vi "Entanglement Table - Read.vi"(7 "QuWire in":refnum<class "QuWire.lvclass">) -> (8 "Mutal Information Table":dbl[][](array[numeric]))   [LabVIEW 2020]
uses:
  QuSim/QuWire/QuWire.lvclass
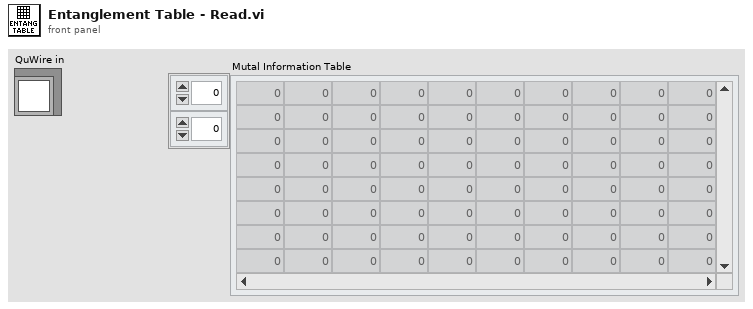
[diagram p1: front panel]
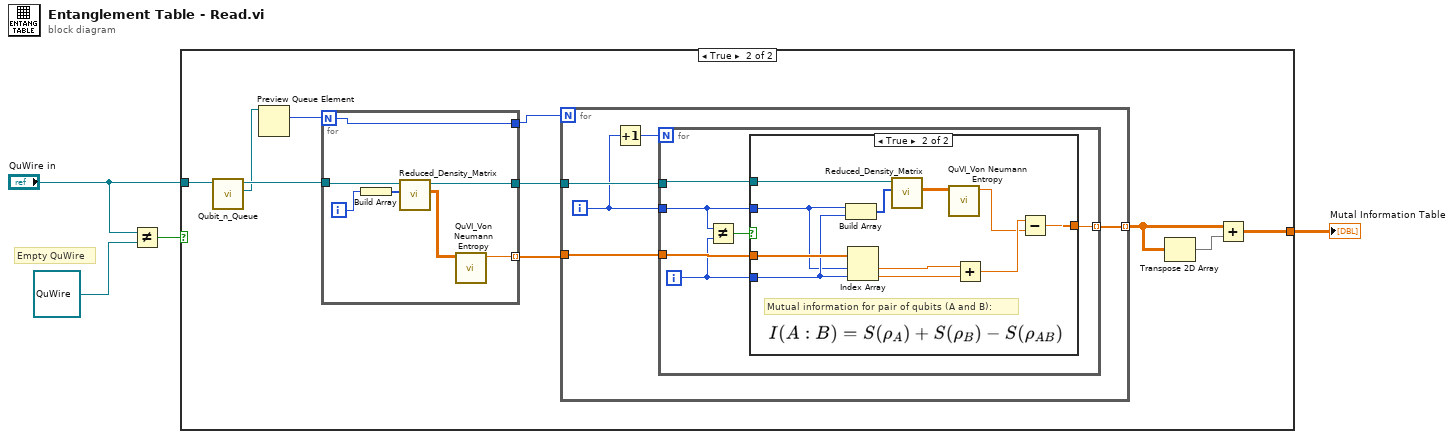
[diagram p0: block diagram]
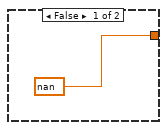
[diagram p3: hidden frame]
diagram:
  # "Empty QuWire"
  n1 = Not Equal?(x="QuWire in", y=refnum<class "QuWire.lvclass"> refnum ("QuWire in")) -> (x != y?=w2:bool)
  n2 = case shown="True" w2 {
    tunnel: "QuWire in" -> [_ w5]
    tunnel: [_ w6] -> w1
    frame False {
    }
    frame True {
      n3 = call "Qubit_n_Queue.vi"("QuWire in"=w5) -> ("Qubit n"=w7:refnum<queue>, "QuWire out"=w9:refnum<class "QuWire.lvclass">)  [unwired: 8 in, 1 out]
      n4 = Preview Queue Element(queue=w7) -> (element=w8:i32)  [unwired: 2 in, 3 out]
      n5 = for {
        N: w8 -> [w17]
        tunnel: w9 -> [w19]
        tunnel: [w18] -> w10
        tunnel: [w17] -> w11
        tunnel: [w15] -> w12 mode=indexing
        i -> [w21]
        n6 = Build Array(w21) -> (w20:i32[])
        n7 = call "Reduced_Density_Matrix.vi"("Qubits to Keep"=w20, "QuWire in"=w19) -> ("Reduced Density Matrix"=w16:cdb[][], "QuWire out"=w18:refnum<class "QuWire.lvclass">)  [unwired: 6 in, 2 out]
        n8 = call "QuVI_Von Neumann Entropy.vi"("Density matrix"=w16) -> ("Von Neumann entropy"=w15:dbl)  [unwired: 10 in]
      }
      n9 = for {
        N: w11 -> [_]
        tunnel: w10 -> [w26]
        tunnel: w12 -> [w25]
        tunnel: [w24] -> w14 mode=indexing
        i -> [w23]
        n10 = Increment(x=w23) -> (x+1=w22:i32)
        n11 = for {
          N: w22 -> [_]
          tunnel: w26 -> [w32]
          tunnel: w25 -> [w31]
          tunnel: [w30] -> w24 mode=indexing
          tunnel: w23 -> [w27]
          i -> [w28]
          n12 = Not Equal?(x=w27, y=w28) -> (x != y?=w29:bool)
          n13 = case shown="True" w29 {
            tunnel: w32 -> [_ w43]
            tunnel: w31 -> [_ w41]
            tunnel: [nan w36] -> w30
            tunnel: w28 -> [_ w35]
            tunnel: w27 -> [_ w34]
            frame False {
            }
            frame True {
              # "Mutual information for pair of qubits (A and B):"
              n14 = Build Array(w34, w35) -> (w44:i32[])
              n15 = Index Array(array=w41, index #1=w34, index #2=w35) -> (element #1=w40:dbl, element #2=w39:dbl)
              n16 = call "Reduced_Density_Matrix.vi"("Qubits to Keep"=w44, "QuWire in"=w43) -> ("Reduced Density Matrix"=w42:cdb[][])  [unwired: 6 in, 3 out]
              n17 = call "QuVI_Von Neumann Entropy.vi"("Density matrix"=w42) -> ("Von Neumann entropy"=w37:dbl)  [unwired: 10 in]
              n18 = Add(x=w40, y=w39) -> (x+y=w38:dbl)
              n19 = Subtract(x=w38, y=w37) -> (x-y=w36:dbl)
            }
          }
        }
      }
      n20 = Transpose 2D Array(2D array=w14) -> (transposed array=w13:dbl[][])
      n21 = Add(x=w14, y=w13) -> (x+y=w6:dbl[][])
    }
  }
  "Mutal Information Table" <- w1
